vi "Write UserEventDLCommand.vi"(8 "error in (no error)":errorcluster caption="entrée d'erreur (pas d'erreur)", 10 "UserEventDLCommand":refnum<user-event>, 11 "DelayLine en entrée":refnum<class "DelayLine.lvclass">) -> (0 "error out":errorcluster caption="sortie d'erreur", 3 "DelayLine en sortie":refnum<class "DelayLine.lvclass">)   [LabVIEW 2015]
uses:
  DelayLine.lvclass
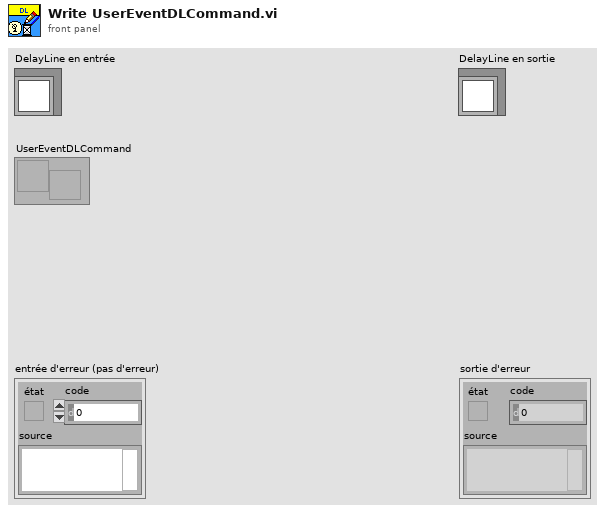
[diagram p1: front panel]
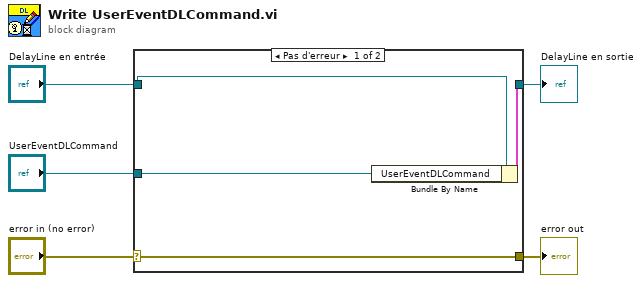
[diagram p0: block diagram]
diagram:
  n1 = case shown="Pas d'erreur" "error in (no error)" {
    selector: "error in (no error)" -> [w9 w10]
    tunnel: [w9 w10] -> w4
    tunnel: [w7 w11] -> w2
    tunnel: "DelayLine en entrée" -> [w8 w11]
    tunnel: "UserEventDLCommand" -> [w6 _]
    frame No Error {
      n2 = Bundle By Name(cluster=w8, "UserEventDLCommand"=w6) -> (w7:cluster{})
    }
    frame Error {
    }
  }
  "error out" <- w4
  "DelayLine en sortie" <- w2
